vi "OpenG Array Sort XNode 2D.vi"(6 "Column/Row to Sort By":u32, 8 "Sort By in":enum16{"row", "column"}(ring), 9 "Order":enum16{"ascending", "descending"}(ring), 11 "Array in":u8[][](array[numeric])) -> (0 "Sort By out":enum16{"row", "column"}(ring), 1 "Index Out of Range?":bool, 2 "Sorted Pointers":i32[](array[numeric]), 3 "Sorted Array out":u8[][](array[numeric]))   [LabVIEW 2018]
doc: "This polymorphic VI sorts a 2D array of numerics or strings, regardless of the array size. You can specify whether to sort by column or row, which column or row to sort by, and whether to sort in ascending or descending order. You also can specify a secondary row or column to sort by."
panel:
  # "[OpenG VI Tags] ***Do Not Remove***\n\nSVN Revision = 990\nSVN Revision Date = 2009-07-18 07:14:13 -0700 (Sat, 18 Jul 2009)\nPackage = oglib_array-3.0.0-1\nDepends ="
  # "Sort 2D Array\n\nThis VI sorts by row or by column, a 2D array of any size in descending or ascending order based on a column or row whose index you specify.\n\nPlease visit http://www.OpenG.org to learn about the\nOpen Source LabVIEW software movement.\n\nNOTICE -- YOU MUST LEAVE THIS NOTICE IN PLACE.  PER THE TERMS OF THE LICENSE BELOW, YOU MAY SUBLICENSE THIS SOFTWARE \nIN ANY WAY THAT DOES NOT CONFLICT WITH THIS LICENSE.\n\n### BSD License (http://www.opensource.org/licenses/bsd-license.php) Begin ###\n \nCopyright (c) 2002, Jim Kring <jim@jimkring.com>\nCopyright (c) 2002, Cal-Bay Systems, Inc. <info@calbay.com>\n\nAll rights reserved.\n\nRedistribution and use in source and binary forms, with or without modification, are permitted provided that the following conditions are met:\n\n    * Redistributions of source code must retain the above copyright notice, this list of conditions and the following disclaimer.\n    * Redistributions in binary form must reproduce the above copyright notice, this list of conditions and the following disclaimer in the \n       documentation and/or other materials provided with the distribution.\n    * Neither the name of SciWare, James Kring, Inc., nor the names of its contributors may be used to endorse or promote products derived \n       from this software without specific prior written permission.\n\nTHIS SOFTWARE IS PROVIDED BY THE COPYRIGHT HOLDERS AND CONTRIBUTORS \"AS IS\" AND ANY EXPRESS OR IMPLIED WARRANTIES, \nINCLUDING, BUT NOT LIMITED TO, THE IMPLIED WARRANTIES OF MERCHANTABILITY AND FITNESS FOR A PARTICULAR PURPOSE ARE \nDISCLAIMED. IN NO EVENT SHALL THE COPYRIGHT OWNER OR CONTRIBUTORS BE LIABLE FOR ANY DIRECT, INDIRECT, INCIDENTAL,\n SPECIAL, EXEMPLARY, OR CONSEQUENTIAL DAMAGES (INCLUDING, BUT NOT LIMITED TO, PROCUREMENT OF SUBSTITUTE GOODS OR \nSERVICES; LOSS OF USE, DATA, OR PROFITS; OR BUSINESS INTERRUPTION) HOWEVER CAUSED AND ON ANY THEORY OF LIABILITY, \nWHETHER IN CONTRACT, STRICT LIABILITY, OR TORT (INCLUDING NEGLIGENCE OR OTHERWISE) ARISING IN ANY WAY OUT OF THE USE \nOF THIS SOFTWARE, EVEN IF ADVISED OF THE POSSIBILITY OF SUCH DAMAGE.\n\n### BSD License End ###"
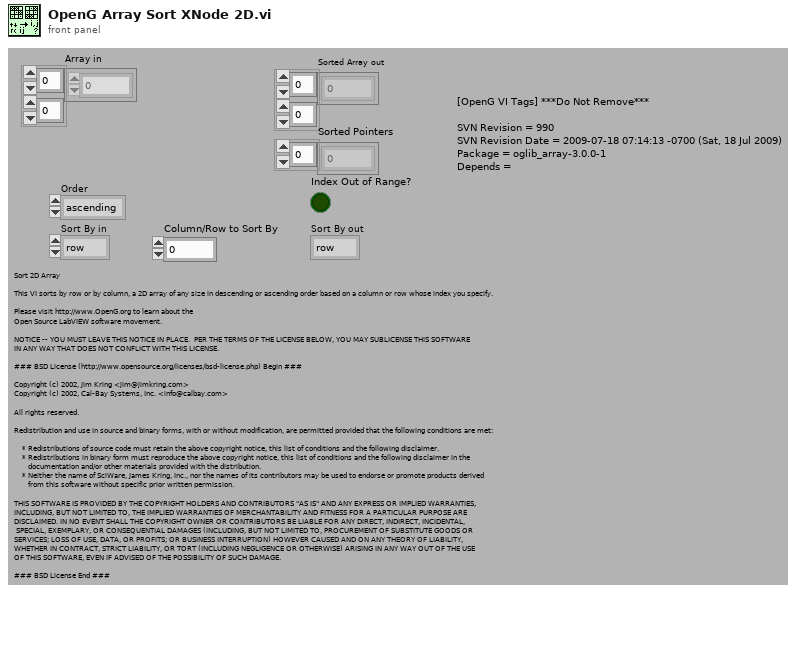
[diagram p1: front panel]
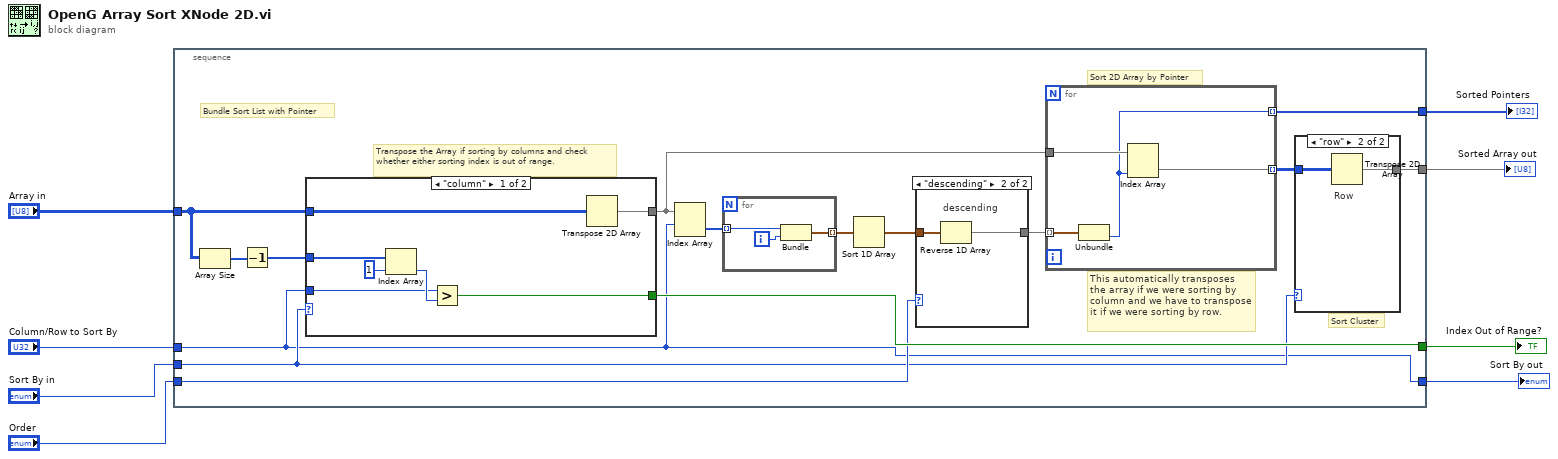
[diagram p0: block diagram]
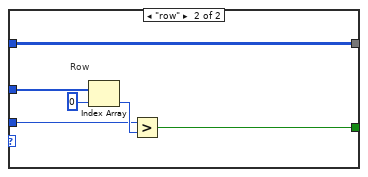
[diagram p4: hidden frame]
diagram:
  n1 = stacked-sequence {
    tunnel: [w21] -> w8
    tunnel: "Array in" -> [w20]
    tunnel: [w18] -> w6
    tunnel: "Column/Row to Sort By" -> [w9]
    tunnel: "Order" -> [w16]
    tunnel: [w11] -> w3
    tunnel: "Sort By in" -> [w10]
    tunnel: [w9] -> w1
    frame #0 {
      # "Sort 2D Array by Pointer"
      # "Sort Cluster"
      # "This automatically transposes the array if we were sorting by column and we have to transpose it if we were sorting by row."
      # "Bundle Sort List with Pointer"
      # "Transpose the Array if sorting by columns and check whether either sorting index is out of range."
      n2 = Array Size(array=w20) -> (size(s)=w19:i32[])
      n3 = Decrement(x=w19) -> (x-1=w17:i32[])
      n4 = case shown="\"column\"" w10 {
        tunnel: w20 -> [w43 w49]
        tunnel: [w42 w49] -> w23
        tunnel: w17 -> [w41 w46]
        tunnel: [w37 w44] -> w18
        tunnel: w9 -> [w38 w45]
        frame "column" {
          n5 = Index Array(array=w41, index=1 ("Index")) -> (element=w39:i32)
          n6 = Greater?(x=w38, y=w39) -> (0:w37:bool)
          n7 = Transpose 2D Array(2D array=w43) -> (transposed array=w42:u8[][])
        }
        frame "row" {
          # "Row"
          n8 = Index Array(array=w46, index=0 ("Index")) -> (element=w48:i32)
          n9 = Greater?(x=w45, y=w48) -> (0:w44:bool)
        }
      }
      n10 = Index Array(array=w23, index (row)=w9) -> (element=w14:u8[])  [unwired: 1 in]
      n11 = for {
        tunnel: w14 -> [w26] mode=indexing
        tunnel: [w24] -> w13 mode=indexing
        i -> [w25]
        n12 = Bundle("Numeric"=w26, w25) -> (w24:cluster{"Numeric":u8, i32})  [unwired: 1 out]
      }
      n13 = Sort 1D Array(array=w13) -> (sorted array=w12:cluster{"Numeric":u8, i32}[])
      n14 = case shown="\"descending\"" w16 {
        tunnel: [w27 w28] -> w15
        tunnel: w12 -> [w27 w29]
        frame "ascending", Default {
        }
        frame "descending" {
          # "descending"
          n15 = Reverse 1D Array(array=w29) -> (reversed array=w28:cluster{"Numeric":u8, i32}[])
        }
      }
      n16 = for {
        tunnel: w15 -> [w36] mode=indexing
        tunnel: w23 -> [w35]
        tunnel: [w34] -> w22 mode=indexing
        tunnel: [w33] -> w11 mode=indexing
        n17 = Unbundle(w36) -> (w33:i32)  [unwired: 1 out]
        n18 = Index Array(array=w35, index (col)=w33) -> (element=w34:u8[])  [unwired: 1 in]
      }
      n19 = case shown="\"row\"" w10 {
        tunnel: w22 -> [w30 w32]
        tunnel: [w30 w31] -> w21
        frame "column" {
        }
        frame "row" {
          # "Row"
          n20 = Transpose 2D Array(2D array=w32) -> (transposed array=w31:u8[][])
        }
      }
    }
  }
  "Sorted Array out" <- w8
  "Index Out of Range?" <- w6
  "Sorted Pointers" <- w3
  "Sort By out" <- w1
